vi "PieChart-algo.vi"(7 "Defect Names":string[](array[string]), 8 "error in (no error)":errorcluster, 10 "Array Of Values":dbl[](array[numeric])=[0.0, 0.0, 0.0, 0.0, 0.0, 0.0, 0.0], 11 "Colors":u32[](array[colorbox])) -> (0 "error out":errorcluster, 2 "Lable":picture, 3 "Pie":picture)   [LabVIEW 2019, in "Zen Analytics.lvlib" / "Zen Analytics.lvclass"]
uses:
  Zen Analytics.lvclass
  <vilib>/Utility/miscctls.llb/LVBoundsTypeDef.ctl
panel:
  in  "Defect Statistics":refnum<vi>
  out "Report Values":string[][](array[string])
types:
  T1 = typedef "LVBoundsTypeDef.ctl" = cluster{"Width":u32, "Height":u32}
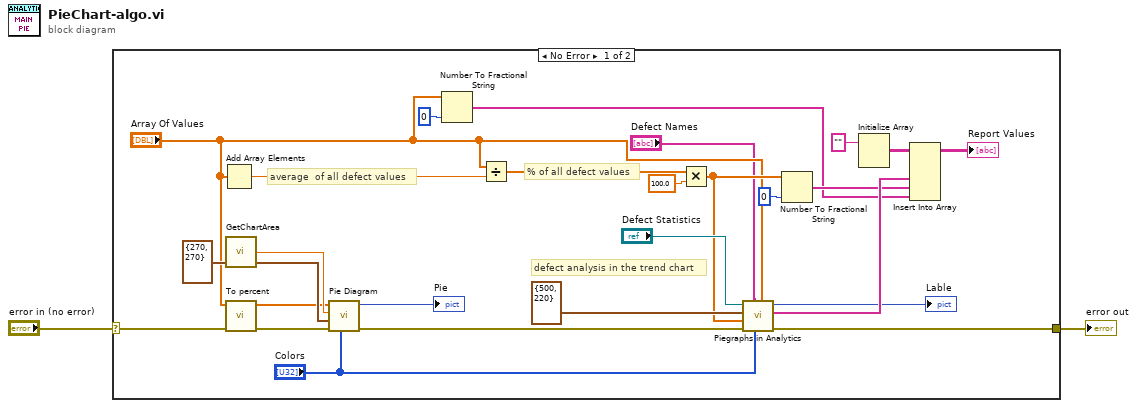
[diagram p0: block diagram]
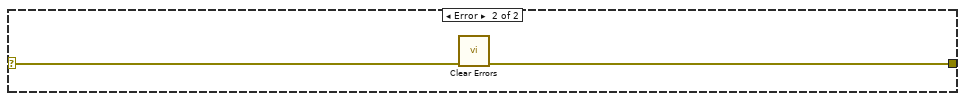
[diagram p2: hidden frame]
diagram:
  n1 = case shown="No Error" "error in (no error)" {
    selector: "error in (no error)" -> [w9 w31]
    tunnel: [w10 w30] -> w1
    frame No Error {
      # "defect analysis in the trend chart"
      # "average  of all defect values"
      # "% of all defect values"
      n2 = Add Array Elements(numeric array="Array Of Values") -> (sum=w18:dbl)
      n3 = call "GetChartArea.vi"("Draw Area Size"=T1 {"Width"=270, "Height"=270} ("Draw Area Size 2")) -> ("Chart Area Size"=w27:cluster{"Width":dbl, "Height":dbl}, "Height"=w26:dbl)  [unwired: 3 in]
      n4 = call "To percent.vi"("error in (no error)"=w9, "I/p"="Array Of Values") -> ("error out"=w6:errorcluster, "O/p"=w23:dbl[])  [unwired: 8 in]
      n5 = call "Pie Diagram.vi"("Array"="Colors", "error in (no error)"=w6, "Chart Area Size"=w27, "Height"=w26, "Values"=w23) -> ("error out"=w7:errorcluster, "new picture"=→"Pie":picture)  [unwired: 5 in]
      n6 = Number To Fractional String(number="Array Of Values", precision (6)=i16 0) -> (F-format string=w12:string[])  [unwired: 2 in]
      n7 = Divide(x="Array Of Values", y=w18) -> (x/y=w22:dbl[])
      n8 = Multiply(x=w22, y=100.0) -> (x*y=w17:dbl[])
      n9 = call "Piegraphs in Analytics.vi"("values"="Array Of Values", "Colors"="Colors", "Defect Names"="Defect Names", "error in (no error)"=w7, "Defect Values"=w17, "Draw Area Size"=T1 {"Width"=500, "Height"=220}, "Defect Statistics"="Defect Statistics") -> ("error out"=w10:errorcluster, "Names with %  values"=w14:string[], "Labels"=→"Lable":picture)  [unwired: 2 in]
      n10 = Number To Fractional String(number=w17, precision (6)=i16 0) -> (F-format string=w13:string[])  [unwired: 2 in]
      n11 = Initialize Array("") -> (w15:string[][])  [unwired: 2 in]
      n12 = Insert Into Array(array=w15, new element #1=w14, new element #2=w13, new element #3=w12) -> (→"Report Values":string[][])  [unwired: 2 in]
    }
    frame Error {
      n13 = call <vilib>:"Clear Errors.vi"("error in (no error)"=w31) -> ("error out"=w30:errorcluster)  [unwired: 5 in, 1 out]
    }
  }
  "error out" <- w1
